vi "SpreadsheetStorage.vi"() -> ()   [LabVIEW 2015]
uses:
  <vilib>/Utility/file.llb/Write Delimited Spreadsheet (DBL).vi
panel:
  in  "Waveform Parameters":T1
  in  "Digitizing Parameters":T2
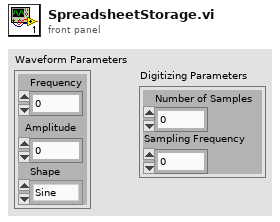
[diagram p1: front panel]
types:
  T1 = cluster{"Frequency":i32, "Amplitude":i32, "Shape":enum16{"Sine", "Cosine", "LinRamp", "Square", "SineCosine"}}
  T2 = cluster{"Number of Samples":i32, "Sampling Frequency":i32}
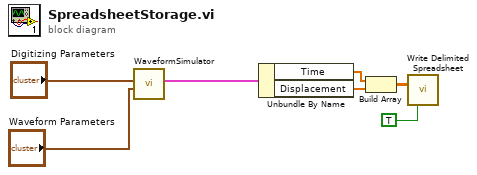
[diagram p0: block diagram]
diagram:
  n1 = call "WaveformSimulator.vi"("Waveform Parameters"="Waveform Parameters", "Digitizing Parameters"="Digitizing Parameters") -> ("Waveform Output"=w5:cluster{"Time":dbl[], "Displacement":dbl[]})  [unwired: 9 in]
  n2 = Unbundle By Name(w5) -> ("Time"=w3:dbl[], "Displacement"=w2:dbl[])
  n3 = Build Array(w3, w2) -> (w1:dbl[][])
  n4 = call-poly <vilib>:"Write Delimited Spreadsheet.vi"("2D data"=w1, "transpose? (F)"=TRUE) -> ()  [unwired: 12 in, 2 out]
